vi "DisableControls.vi"(7 "BusIndex":i32, 8 "Error In":errorcluster[](array[cluster]), 11 "Bus in":refnum<class "Bus.lvclass">) -> (0 "Error Out":errorcluster[](array[cluster]), 3 "Bus out":refnum<class "Bus.lvclass">)   [LabVIEW 2018]
doc: "This VI filters the INI files using the PluginType the applicaitons currently has running."
uses:
  NistPluggableModules/BusClass/Bus.lvclass
  NistPluggableModules/BusClass/Bus.lvclass/Bus.ctl
  NistPluggableModules/TestClass/Test.lvclass/Test.ctl
  NistPluggableModules/BusClass/Accessors/Read Test.vi
  NistPluggableModules/TestClass/Accessors/Read PluginPathArray.vi
  NistPluggableModules/TestClass/Accessors/Write PluginPathArray.vi
  NistPluggableModules/BusClass/Accessors/Write Test.vi
  NistPluggableModules/TestClass/Test.lvclass
  <userlib>/NIST/NISTErrorLib/NISTErrorLib.lvlib
panel:
  out "logical OR":bool
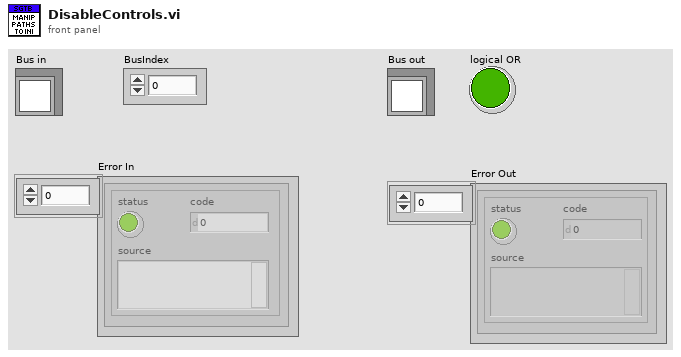
[diagram p1: front panel]
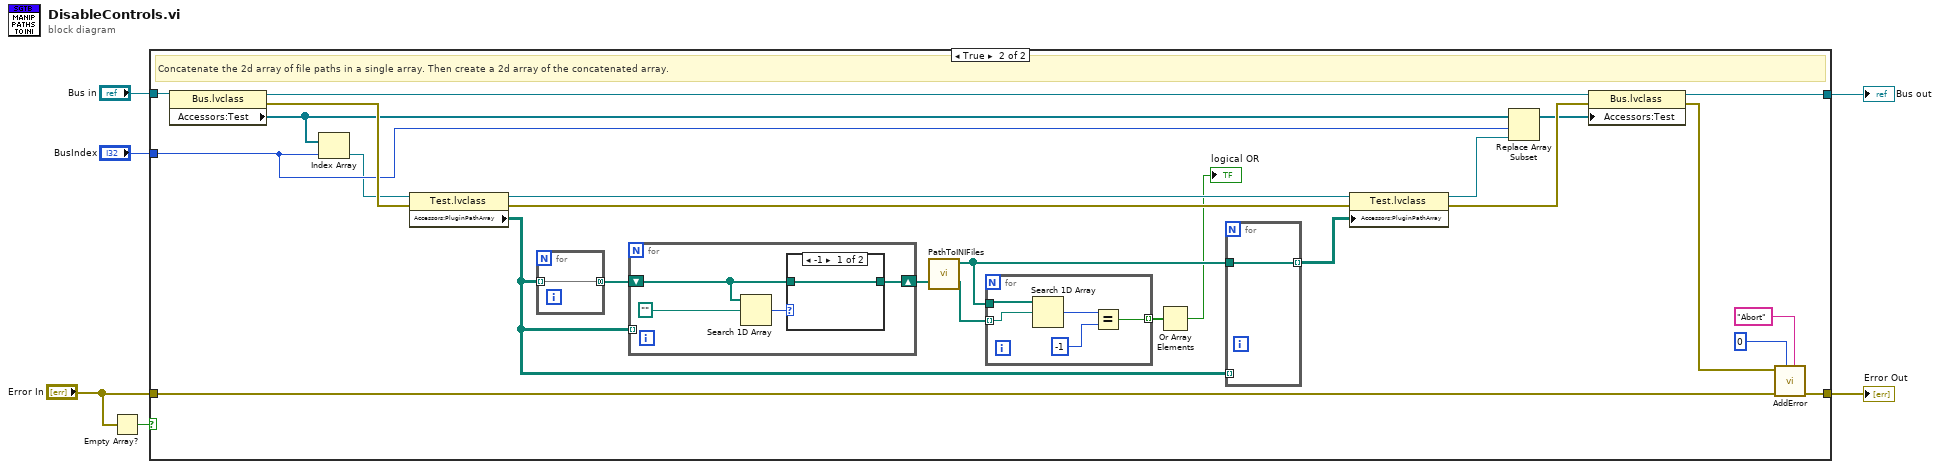
[diagram p0: block diagram]
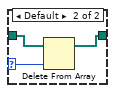
[diagram p3: hidden frame]
diagram:
  n1 = Empty Array?(array="Error In") -> (empty?=w6:bool)
  n2 = case shown="True" w6 {
    tunnel: "Error In" -> [w7 w22]
    tunnel: "Bus in" -> [w8 w32]
    tunnel: [w8 w30] -> w4
    tunnel: [w7 w27] -> w1
    tunnel: "BusIndex" -> [_ w19]
    frame False {
      # "If an error occurs passes the error through and does nothing."
    }
    frame True {
      # "Concatenate the 2d array of file paths in a single array. Then create a 2d array of the concatenated array."
      n3 = property class="Bus.lvclass"(reference=w32) -> (reference out=w31:refnum<class "Bus.lvclass">, error out=w25:errorcluster, "Accessors:Test"=w17:refnum<class "Test.lvclass">[])  [unwired: 1 in]
      n4 = Index Array(array=w17, index=w19) -> (element=w16:refnum<class "Test.lvclass">)
      n5 = property class="Test.lvclass"(reference=w16, error in=w25) -> (reference out=w24:refnum<class "Test.lvclass">, error out=w21:errorcluster, "Accessors:PluginPathArray"=w9:path[][])
      n6 = for {
        tunnel: w9 -> [w33] mode=indexing
        tunnel: [w33] -> w11 mode=concatenating
      }
      n7 = for {
        shift-right: [w37] -> w10
        shift-left: w11 -> [w36]
        tunnel: w9 -> [_] mode=indexing
        n8 = Search 1D Array(1D array=w36, element=path "") -> (index of element=w35:i32)  [unwired: 1 in]
        n9 = case shown="-1" w35 {
          selector: w35 -> [_ w39]
          tunnel: w36 -> [w38 w41]
          tunnel: [w38 w40] -> w37
          frame -1 {
          }
          frame Default {
            n10 = Delete From Array(array=w41, index=w39) -> (array with subset deleted=w40:path[])  [unwired: 1 in, 1 out]
          }
        }
      }
      n11 = call "PathToINIFiles.vi"() -> ("IniFilePaths Out"=w14:path[])  [unwired: 11 in]
      n12 = for {
        tunnel: w10 -> [w43] mode=indexing
        tunnel: w14 -> [w46]
        tunnel: [w42] -> w13 mode=indexing
        n13 = Search 1D Array(1D array=w46, element=w43) -> (index of element=w45:i32)  [unwired: 1 in]
        n14 = Equal?(x=w45, y=-1) -> (x = y?=w42:bool)
      }
      n15 = Or Array Elements(Boolean array=w13) -> (logical OR=→"logical OR":bool)
      n16 = for {
        tunnel: w9 -> [_] mode=indexing
        tunnel: [w47] -> w15 mode=indexing
        tunnel: w14 -> [w47]
      }
      n17 = property class="Test.lvclass"(reference=w24, error in=w21, "Accessors:PluginPathArray"=w15) -> (reference out=w20:refnum<class "Test.lvclass">, error out=w23:errorcluster)
      n18 = Replace Array Subset(array=w17, new element=w20, index=w19) -> (w18:refnum<class "Test.lvclass">[])
      n19 = property class="Bus.lvclass"(reference=w31, error in=w23, "Accessors:Test"=w18) -> (reference out=w30:refnum<class "Bus.lvclass">, error out=w26:errorcluster)
      n20 = call <userlib>:"AddError.vi"("Severity"="Abort", "Priority"=u8 0, "ErrorArray"=w22, "error in (no error)"=w26) -> ("ErrorArray"=w27:errorcluster[])  [unwired: 6 in, 1 out]
    }
  }
  "Bus out" <- w4
  "Error Out" <- w1
